vi "car3udpmsg_receivr.vi"() -> ()   [LabVIEW 2020]
panel:
  out "data (bytes string)":string
  out "timestamp":dbl format="%.3f"
  out "receiver_port":u16=16100
  out "receiver_IPv4":string
  out "sender_port":u16=16100
  out "sender_IPv4":string
  out "msg_len":u16=1
  out "msg_type":u8=1
  out "port":u16=16002
  out "IP":string="192.168.1.2"
  in  "stop":bool
  # "on the cRIO: receive and parse messages"
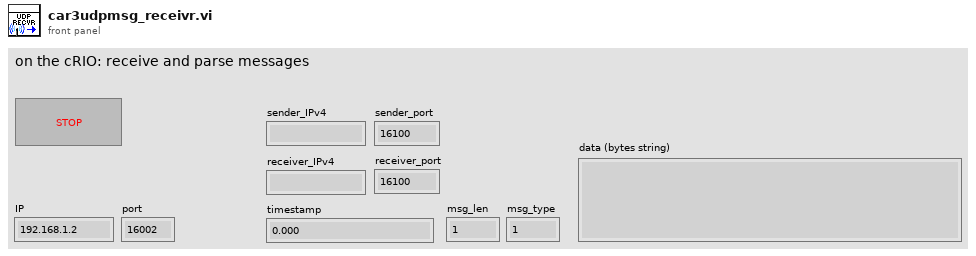
[diagram p1: front panel]
types:
  T1 = cluster{"sender_IPv4":string, "sender_port":u16, "sender_IPv4":string, "sender_port":u16, "sender_port":u16, "timestamp":dbl, "msg_type":u8, "sender_IPv4":string, "cs":u32}
  T2 = cluster{"sender_IPv4":string, "sender_port":u16, "receiver_IPv4":string, "receiver_port":u16, "msg_len":u16, "timestamp":dbl, "msg_type":u8, "data (bytes string)":string, "cs":u32}
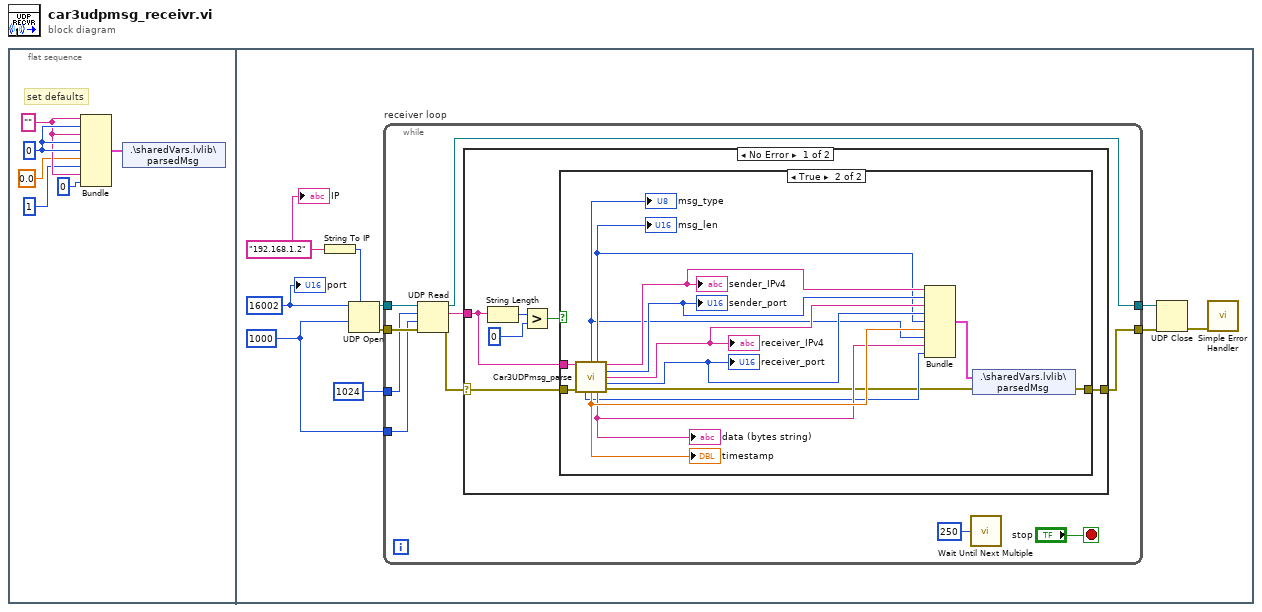
[diagram p0: block diagram]
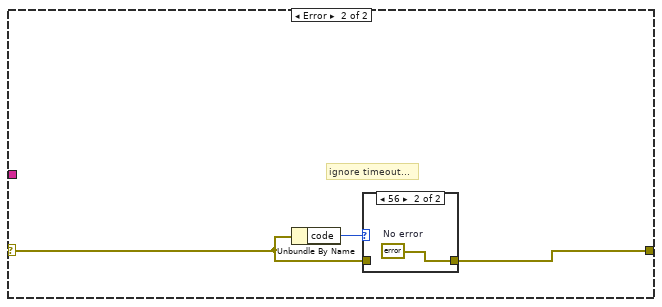
[diagram p3: hidden frame]
diagram:
  n1 = flat-sequence {
    frame #0 {
      w5 = u16 0 ("sender_port")
      w4 = "" ("sender_IPv4")
      # "set defaults"
      n2 = Bundle("sender_IPv4"=w4, "sender_port"=w5, "sender_IPv4"=w4, "sender_port"=w5, "sender_port"=w5, "timestamp"=0.0, "msg_type"=u8 1, "sender_IPv4"=w4, "cs"=u32 0) -> (w6:T1)  [unwired: 1 in]
      n3 = shared-variable ".\\sharedVars.lvlib\\parsedMsg"(w6) -> ()  [unwired: 1 in, 1 out]
    }
    frame #1 {
      w7 = 1000 ("timeout ms (25000)")
      w10 = u16 16002 ("port")
      w11 = "192.168.1.2" ("name")
      n4 = String To IP(1:w11) -> (0:w12:u32)
      n5 = UDP Open(7:w12, 9:w7, 11:w10) -> (port=w14:refnum<k16>, 0:w13:errorcluster)  [unwired: 2 in, 1 out]
      n6 = while "receiver loop" {
        tunnel: [w22] -> w15
        tunnel: w14 -> [w24]
        tunnel: w13 -> [w23]
        tunnel: [w21] -> w9
        tunnel: 1024 ("max size (548)") -> [w20]
        tunnel: w7 -> [w17]
        stop <- "stop" stop-if-true
        n7 = UDP Read(connection ID=w24, max size (548)=w20, timeout ms (25000)=w17, 8:w23) -> (data out=w19:string, error out=w18:errorcluster, 3:w22:refnum<k16>)  [unwired: 2 out]
        n8 = case shown="No Error" w18 {
          selector: w18 -> [w27 w48]
          tunnel: [w32 w49] -> w21
          tunnel: w19 -> [w28 _]
          frame No Error {
            n9 = String Length(string=w28) -> (length=w31:i32)
            n10 = Greater?(x=w31, y=0) -> (0:w29:bool)
            n11 = case shown="True" w29 {
              tunnel: w28 -> [_ w47]
              tunnel: w27 -> [w33 w46]
              tunnel: [w33 w34] -> w32
              frame False {
              }
              frame True {
                n12 = call "Car3UDPmsg_parse.vi"("input (bytes string)"=w47, "error in (no error)"=w46) -> ("msg_type"=w39:u8, "msg_len"=w41:u16, "sender_IPv4"=w45:string, "sender_port"=w44:u16, "receiver_IPv4"=w43:string, "receiver_port"=w42:u16, "cs"=w37:u32, "timestamp"=w40:dbl, "data (bytes string)"=w38:string, "error out"=w35:errorcluster)  [unwired: 4 in]
                "msg_type" <- w39
                "msg_len" <- w41
                "sender_IPv4" <- w45
                "sender_port" <- w44
                "receiver_IPv4" <- w43
                "receiver_port" <- w42
                "timestamp" <- w40
                "data (bytes string)" <- w38
                n13 = Bundle("sender_IPv4"=w45, "sender_port"=w44, "receiver_IPv4"=w43, "receiver_port"=w42, "msg_len"=w41, "timestamp"=w40, "msg_type"=w39, "data (bytes string)"=w38, "cs"=w37) -> (w36:T2)  [unwired: 1 in]
                n14 = shared-variable ".\\sharedVars.lvlib\\parsedMsg"(w36, error in=w35) -> (error out=w34:errorcluster)
              }
            }
          }
          frame Error {
            # "ignore timeout..."
            n15 = Unbundle By Name(w48) -> ("code"=w50:i32)
            n16 = case shown="56" w50 {
              tunnel: w48 -> [w51 _]
              tunnel: [w51 w52] -> w49
              frame Default {
              }
              frame 56 {
                w52 = errorcluster {"status"=FALSE, "code"=0, "source"=""}  # No error
              }
            }
          }
        }
        n17 = call "Wait Until Next Multiple"("Count(mSec)"=u32 250 ("millisecond multiple")) -> ()  [unwired: 1 out]
      }
      n18 = UDP Close(connection ID=w15, 8:w9) -> (error out=w16:errorcluster)  [unwired: 1 out]
      n19 = call <vilib>:"Simple Error Handler.vi"("error in (no error)"=w16) -> ()  [unwired: 4 in, 5 out]
      "IP" <- w11
      "port" <- w10
    }
  }
